vi "GDS_MO_SetEnergy_TEST.vi"() -> ()   [LabVIEW 2015]
uses:
  SES_1.3.1-r26_SES100/dll/MonoHW_Dummy.dll
panel:
  out "x = y?":bool
  out "error out":errorcluster
  out "return type":i8
  out "SPEC:ExpNumber_RQ":dbl
  out "SES:monochromater_SV":dbl
  in  "AEnergy":dbl=5.0
  # "SetEnergy"
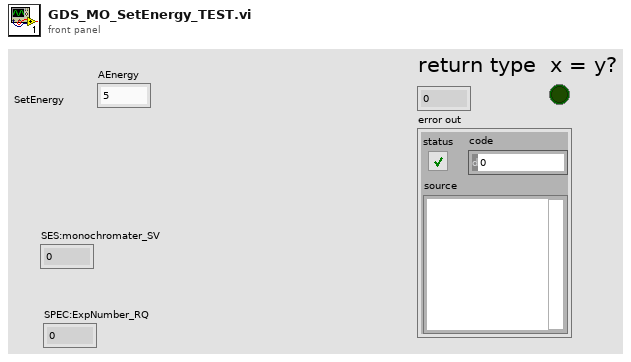
[diagram p1: front panel]
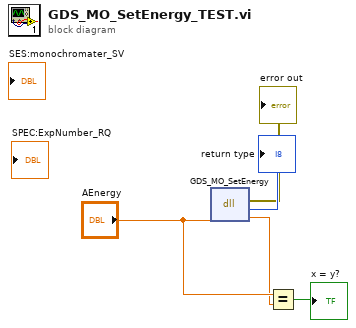
[diagram p0: block diagram]
diagram:
  n1 = dll-call lib="S:/SES_1.3.1-r26_SES100/dll/MonoHW_Dummy.dll" fn="GDS_MO_SetEnergy"("AEnergy"="AEnergy") -> (error out=→"error out":errorcluster, "return type"=→"return type":i8, "AEnergy"=w2:dbl)  [unwired: 3 in, 1 out]
  n2 = Equal?(x="AEnergy", y=w2) -> (x = y?=→"x = y?":bool)
